vi "Withdraw.vi"(8 "file path":path, 9 "Account No.":string, 10 "Amount":string) -> (1 "Output":string)   [LabVIEW 2023]
uses:
  <vilib>/Utility/file.llb/Read Delimited Spreadsheet (string).vi
  <vilib>/Utility/file.llb/Write Delimited Spreadsheet (string).vi
panel:
  # "Output"
  # "Input"
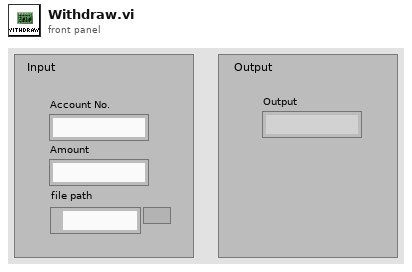
[diagram p1: front panel]
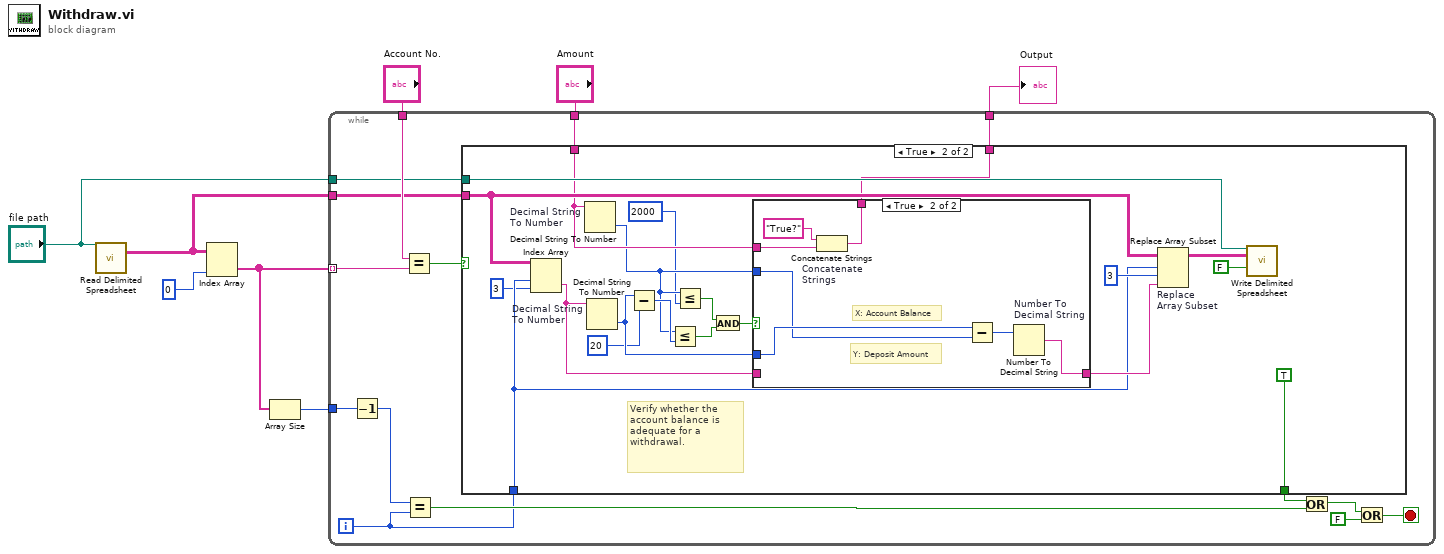
[diagram p0: block diagram]
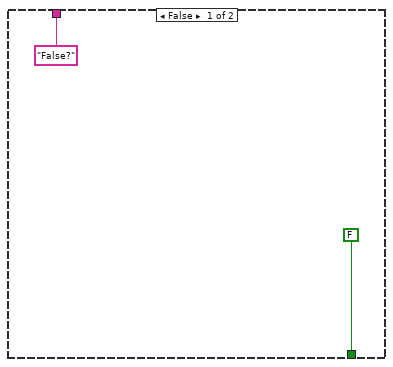
[diagram p2: hidden frame]
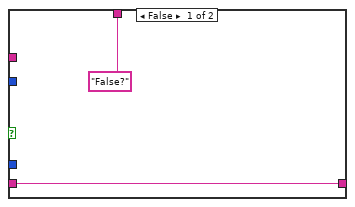
[diagram p3: hidden frame]
diagram:
  n1 = call-poly <vilib>:"Read Delimited Spreadsheet.vi"("file path (dialog if empty)"="file path") -> ("all rows"=w6:string[][])  [unwired: 9 in, 5 out]
  n2 = Index Array "Index Array"(array=w6, index (col)=0 ("index")) -> (element=w7:string[])  [unwired: 1 in]
  n3 = Array Size(array=w7) -> (size(s)=w8:i32)
  n4 = while {
    tunnel: w8 -> [w21]
    tunnel: w7 -> [w17] mode=indexing
    tunnel: w6 -> [w13]
    tunnel: "file path" -> [w12]
    tunnel: "Account No." -> [w16]
    tunnel: "Amount" -> [w11]
    tunnel: [w10] -> w1
    i -> [w15]
    stop <- w23 stop-if-true
    n5 = Decrement(x=w21) -> (x-1=w22:i32)
    n6 = Equal?(x=w16, y=w17) -> (x = y?=w14:bool)
    n7 = Equal?(x=w22, y=w15) -> (x = y?=w18:bool)
    n8 = case shown="True" w14 {
      tunnel: [FALSE TRUE] -> w9
      tunnel: w15 -> [_ w36]
      tunnel: w13 -> [_ w42]
      tunnel: w11 -> [_ w34]
      tunnel: w12 -> [_ w43]
      tunnel: ["False?" w38] -> w10
      frame False {
      }
      frame True {
        # "Verify whether the account balance is adequate for a withdrawal."
        n9 = Index Array "Index Array"(array=w42, index (row)=w36, index (col)=3 ("disabled index (row)")) -> (element=w37:string)
        n10 = Decimal String To Number "Decimal String\nTo Number"(string=w34) -> (number=w30:i32)  [unwired: 2 in, 1 out]
        n11 = Decimal String To Number "Decimal String\nTo Number"(string=w37) -> (number=w33:i32)  [unwired: 2 in, 1 out]
        n12 = Subtract(x=w33, y=20) -> (x-y=w31:i32)
        n13 = Less Or Equal?(x=w30, y=w31) -> (x <= y?=w27:bool)
        n14 = Less Or Equal?(x=w30, y=2000) -> (x <= y?=w26:bool)
        n15 = And(x=w26, y=w27) -> (x .and. y?=w28:bool)
        n16 = case shown="True" w28 {
          tunnel: w30 -> [_ w51]
          tunnel: w33 -> [_ w52]
          tunnel: [w46 w54] -> w39
          tunnel: ["False?" w50] -> w38
          tunnel: w37 -> [w46 _]
          tunnel: w34 -> [_ w48]
          frame False {
          }
          frame True {
            # "Y: Deposit Amount"
            # "X: Account Balance"
            n17 = Concatenate Strings "Concatenate \nStrings"("True?", w48) -> (w50:string)
            n18 = Subtract(x=w52, y=w51) -> (x-y=w53:i32)
            n19 = Number To Decimal String "Number To\nDecimal String"(number=w53) -> (decimal integer string=w54:string)  [unwired: 1 in]
          }
        }
        n20 = Replace Array Subset "Replace \nArray Subset"(array=w42, new element=w39, index (row)=w36, index (col)=3 ("disabled index (col)")) -> (w40:string[][])
        n21 = call-poly <vilib>:"Write Delimited Spreadsheet.vi"("file path (dialog if empty)"=w43, "2D data"=w40, "append to file? (new file:F)"=FALSE) -> ()  [unwired: 11 in, 2 out]
      }
    }
    n22 = Or(x=w9, y=w18) -> (x .or. y?=w19:bool)
    n23 = Or(x=w19, y=FALSE) -> (x .or. y?=w23:bool)
  }
  "Output" <- w1
